vi "Rectangle Comparison.vi"(6 "Line Border":cluster{"Top":dbl, "Bottom":dbl}={"Top"=6.0, "Bottom"=1.0}, 9 "Second":dbl[](array[numeric]), 11 "First":dbl[](array[numeric])) -> (0 "Rect Out":T1 {"Bottom" format="%#_3g"; "Right" format="%#_3g"; "Top" format="%#_3g"; "Left" format="%#_3g"}, 1 "Line Out":T2, 3 "Scores Out":T3)   [LabVIEW 2017, in "VisionSystem.lvlib"]
uses:
  VisionSystem.lvlib
  Cluster_Line.ctl
  Cluster_UI DBL Box.ctl
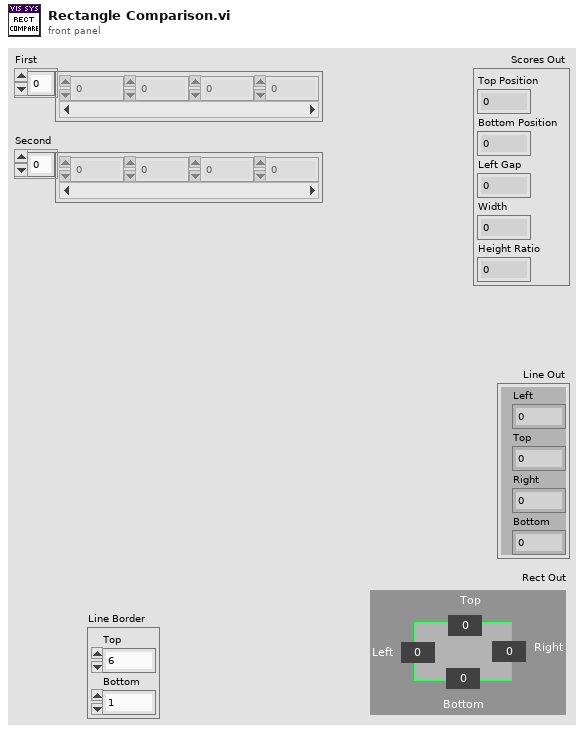
[diagram p1: front panel]
types:
  T1 = typedef "VisionSystem.lvlib/Cluster_UI DBL Box.ctl" = cluster{"Left":dbl, "Top":dbl, "Right":dbl, "Bottom":dbl}
  T2 = typedef "VisionSystem.lvlib/Cluster_Line.ctl" = cluster{"Left":dbl, "Top":dbl, "Right":dbl, "Bottom":dbl}
  T3 = cluster{"Top Position":dbl, "Bottom Position":dbl, "Left Gap":dbl, "Width":dbl, "Height Ratio":dbl}
  T4 = cluster{"[0]":dbl, "[1]":dbl, "[2]":dbl, "[3]":dbl}
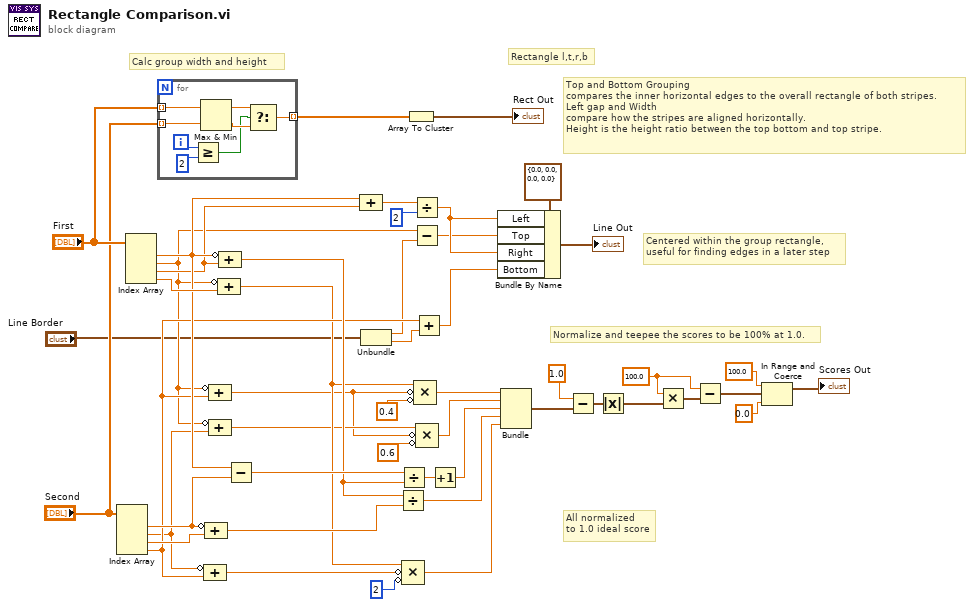
[diagram p0: block diagram]
diagram:
  w21 = 100.0 ("x/y")
  # "Centered within the group rectangle,\nuseful for finding edges in a later step"
  # "All normalized\nto 1.0 ideal score"
  # "Normalize and teepee the scores to be 100% at 1.0."
  # "Top and Bottom Grouping\ncompares the inner horizontal edges to the overall rectangle of both stripes.\nLeft gap and Width\ncompare how the stripes are aligned horizontally.\nHeight is the height ratio between the top bottom and top stripe."
  # "Calc group width and height"
  # "Rectangle l,t,r,b"
  n1 = Index Array(array="Second") -> (element #1=w45:dbl, element #2=w11:dbl, element #3=w48:dbl, element #4=w13:dbl)  [unwired: 4 in]
  n2 = Index Array(array="First") -> (element #1=w37:dbl, element #2=w10:dbl, element #3=w36:dbl, element #4=w38:dbl)  [unwired: 4 in]
  n3 = for {
    tunnel: "First" -> [w56] mode=indexing
    tunnel: "Second" -> [w55] mode=indexing
    tunnel: [w49] -> w28 mode=indexing
    i -> [w53]
    n4 = Greater Or Equal?(x=w53, y=2) -> (x >= y?=w50:bool)
    n5 = Max & Min(x=w56, y=w55) -> (max(x,y)=w52:dbl, min(x,y)=w51:dbl)
    n6 = Select(t=w52, s=w50, f=w51) -> (s? t:f=w49:dbl)
  }
  n7 = Compound Arithmetic op=ADD(invert w11, w13) -> (w46:dbl)
  n8 = Compound Arithmetic op=ADD(invert w45, w48) -> (w47:dbl)
  n9 = Compound Arithmetic op=ADD(invert w10, w13) -> (w8:dbl)
  n10 = Compound Arithmetic op=ADD(invert w10, w11) -> (w9:dbl)
  n11 = Compound Arithmetic op=ADD(invert w10, w38) -> (w12:dbl)
  n12 = Compound Arithmetic op=ADD(invert w37, w36) -> (w43:dbl)
  n13 = Subtract(x=w37, y=w45) -> (x-y=w44:dbl)
  n14 = Compound Arithmetic op=ADD(w37, w36) -> (w35:dbl)
  n15 = Unbundle("Line Border") -> ("Top"=w2:dbl, "Bottom"=w3:dbl)
  n16 = Divide(x=w43, y=w47) -> (x/y=w41:dbl)
  n17 = Divide(x=w44, y=w43) -> (x/y=w39:dbl)
  n18 = Compound Arithmetic op=MULTIPLY(w12, invert w46, invert 2) -> (w40:dbl)
  n19 = Array To Cluster(array=w28) -> (cluster=→"Rect Out":T4)
  n20 = Divide(x=w35, y=2) -> (x/y=w34:dbl)
  n21 = Subtract(x=w10, y=w2) -> (x-y=w32:dbl)
  n22 = Add(x=w13, y=w3) -> (x+y=w26:dbl)
  n23 = Compound Arithmetic op=MULTIPLY(w12, invert w8, invert 0.4 ("y")) -> (w42:dbl)
  n24 = Compound Arithmetic op=MULTIPLY(w9, invert w8, invert 0.6 ("y")) -> (w7:dbl)
  n25 = Increment(x=w39) -> (x+1=w25:dbl)
  n26 = Bundle By Name(cluster=T2 {"Left"=0.0, "Top"=0.0, "Right"=0.0, "Bottom"=0.0} ("Line Out"), "Left"=w34, "Top"=w32, "Right"=w34, "Bottom"=w26) -> (→"Line Out":T2)
  n27 = Bundle(w42, w7, w25, w41, w40) -> (w15:cluster{dbl, dbl, dbl, dbl, dbl})  [unwired: 1 in]
  n28 = Subtract(x=1.0 ("y"), y=w15) -> (x-y=w19:cluster{dbl, dbl, dbl, dbl, dbl})
  n29 = Absolute Value(x=w19) -> (abs(x)=w22:cluster{dbl, dbl, dbl, dbl, dbl})
  n30 = Multiply(x=w21, y=w22) -> (x*y=w23:cluster{dbl, dbl, dbl, dbl, dbl})
  n31 = Subtract(x=w21, y=w23) -> (x-y=w18:cluster{dbl, dbl, dbl, dbl, dbl})
  n32 = In Range and Coerce(upper limit=100.0, x=w18, lower limit=0.0) -> (coerced(x)=→"Scores Out":cluster{dbl, dbl, dbl, dbl, dbl})  [unwired: 1 out]
